vi "Servo_init.vi"(2 "error in (no error)":errorcluster) -> (0 "error out":errorcluster)   [LabVIEW 2009, in "Servo.lvlib"]
uses:
  Servo.lvlib
  <vilib>/Utility/config.llb/Read Key (Double).vi
  <vilib>/Utility/config.llb/NI_LVConfig.lvlib
panel:
  out "appended path":path
  out "Array":T1(array[cluster])
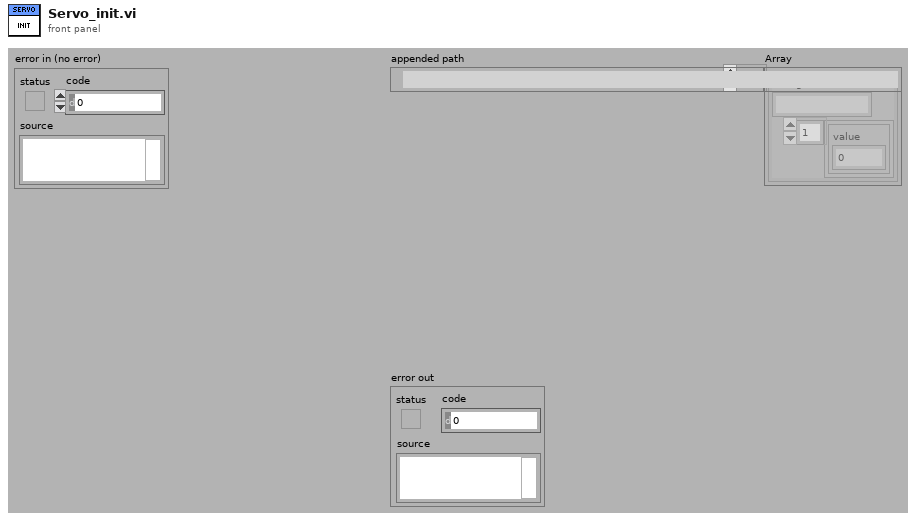
[diagram p1: front panel]
types:
  T1 = cluster{"String":string, cluster{"value":dbl}[]}[]
  T2 = typedef "NI_LVConfig.lvlib/Config Data RefNum.ctl" = refnum<k1>
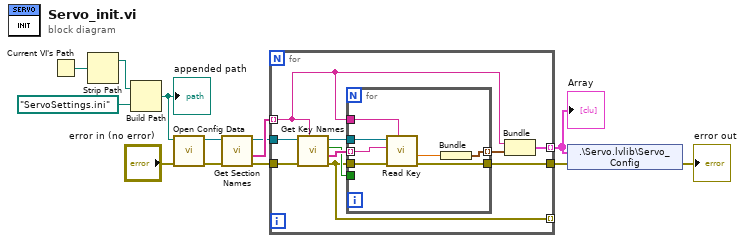
[diagram p0: block diagram]
diagram:
  n1 = Current VI's Path() -> (path=w5:path)
  n2 = Strip Path(path=w5) -> (stripped path=w4:path)  [unwired: 1 out]
  n3 = Build Path(base path=w4, name or relative path=path "ServoSettings.ini" ("configuration file path")) -> (appended path=w6:path)
  "appended path" <- w6
  n4 = call <vilib>:"Open Config Data.vi"("error in (no error)"="error in (no error)", "configuration file path"=w6) -> ("error out"=w12:errorcluster, "refnum"=w13:T2)  [unwired: 7 in, 1 out]
  n5 = call <vilib>:"Get Section Names.vi"("error in (no error)"=w12, "refnum"=w13) -> ("error out"=w9:errorcluster, "section names"=w11:string[], "refnum out"=w10:T2)  [unwired: 7 in]
  n6 = for {
    tunnel: w11 -> [w17] mode=indexing
    tunnel: w10 -> [w20]
    tunnel: w9 -> [w19]
    tunnel: [w18] -> w3
    tunnel: [w16] -> w8 mode=indexing
    tunnel: [w14] -> _ mode=indexing
    n7 = call <vilib>:"Get Key Names.vi"("section"=w17, "error in (no error)"=w19, "refnum"=w20) -> ("error out"=w14:errorcluster, "key names"=w23:string[], "section exists?"=w21:bool, "refnum out"=w22:T2)  [unwired: 5 in]
    n8 = for {
      tunnel: w23 -> [w27] mode=indexing
      tunnel: w14 -> [w30]
      tunnel: w22 -> [w29]
      tunnel: [w28] -> w18
      tunnel: w21 -> [_]
      tunnel: w17 -> [w26]
      tunnel: [w24] -> w15 mode=indexing
      n9 = call-poly <vilib>:"Read Key.vi"("section"=w26, "error in (no error)"=w30, "key"=w27, "refnum"=w29) -> ("error out"=w28:errorcluster, "value"=w25:dbl)  [unwired: 4 in, 2 out]
      n10 = Bundle("value"=w25) -> (w24:cluster{"value":dbl})  [unwired: 1 in]
    }
    n11 = Bundle("String"=w17, w15) -> (w16:cluster{"String":string, cluster{"value":dbl}[]})  [unwired: 1 in]
  }
  "Array" <- w8
  n12 = shared-variable ".\\Servo.lvlib\\Servo_Config"(w8, error in=w3) -> (error out=→"error out":errorcluster)
